vi "EndTestCalled.vi"(1 "FakeTestListener In":refnum<class "FakeTestListener.lvclass">) -> (0 "EndTest Called":bool)   [LabVIEW 2017, in "TestResultTest.lvlib" / "Support.lvlib" / "FakeTestListener.lvclass"]
uses:
  FakeTestListener.lvclass
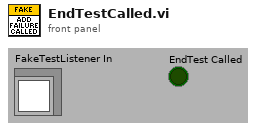
[diagram p1: front panel]
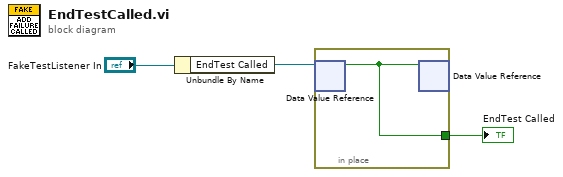
[diagram p0: block diagram]
diagram:
  n1 = Unbundle By Name("FakeTestListener In") -> ("EndTest Called"=w2:refnum<data-value>)
  n2 = in-place {
    in-place-border: [w4] -> w1
    n3 = in-place-dvr #1(w2) -> (w4:bool)  [unwired: 1 out]
    n4 = in-place-dvr #1(w4) -> ()  [unwired: 2 out]
  }
  "EndTest Called" <- w1
